vi "Valor PID.vi"(7 "PI":cluster{"P":dbl, "I":dbl}, 8 "Current":dbl, 11 "Target":dbl) -> (2 "Output":dbl, 4 "Error":dbl)   [LabVIEW 2016]
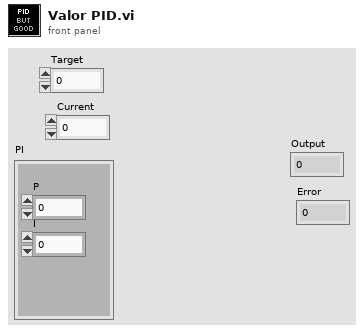
[diagram p1: front panel]
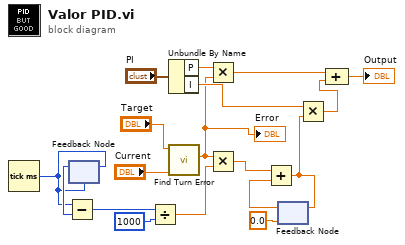
[diagram p0: block diagram]
diagram:
  n1 = Tick Count (ms)() -> (millisecond timer value=w11:u32)
  n2 = feedback #1(w11) -> (w12:u32)
  n3 = Subtract(x=w11, y=w12) -> (x-y=w10:u32)
  n4 = feedback-in #1(w11) -> ()
  n5 = Divide(x=w10, y=u32 1000) -> (x/y=w8:dbl)
  n6 = Unbundle By Name("PI") -> ("P"=w13:dbl, "I"=w3:dbl)
  n7 = call "Find Turn Error.vi"("Target Angle"="Target", "Current Angle"="Current") -> ("Error"=w1:dbl)  [unwired: 7 in]
  "Error" <- w1
  n8 = Multiply(x=w13, y=w1) -> (x*y=w15:dbl)
  n9 = Multiply(x=w1, y=w8) -> (x*y=w7:dbl)
  n10 = feedback #2(0.0) -> (w5:dbl)
  n11 = Add(x=w7, y=w5) -> (x+y=w4:dbl)
  n12 = feedback-in #2(w4) -> ()
  n13 = Multiply(x=w3, y=w4) -> (x*y=w2:dbl)
  n14 = Compound Arithmetic op=ADD(w15, w2) -> (→"Output":dbl)
